vi "AssembleBLMultiplotScript-UandTI-CPPPNG.vi"(1 "Final Title":string, 2 "Spectra?":bool, 4 "Zref":dbl, 8 "Scale":dbl, 9 "BL Targets":T1[](array[typedef]) {"n" min=0.02 max=0.5 step=0.01 format="%.2f"}) -> (20 "gnuplotOut":string)   [LabVIEW 2021]
uses:
  BLTarget.ctl
  Results_plotter_Global.vi
panel:
  # "Currently displayed BL Target velocity profile will be overlaid"
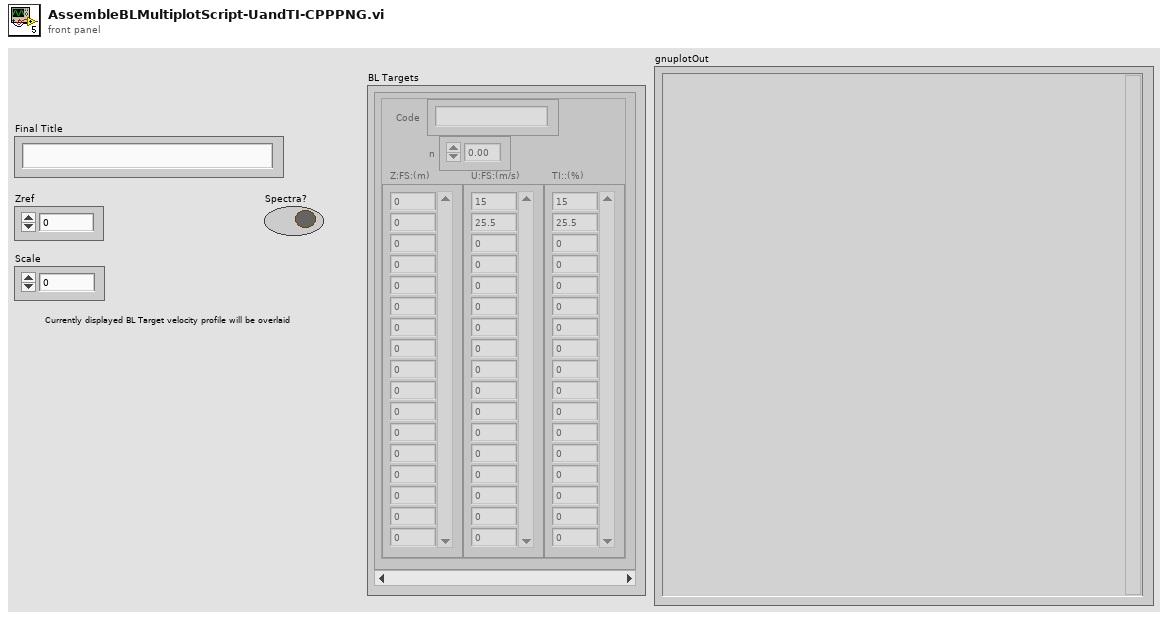
[diagram p1: front panel]
types:
  T1 = typedef "BLTarget.ctl" = cluster{"Code":string, "n":dbl, "Z:FS:(m)":dbl[], "U:FS:(m/s)":dbl[], "TI::(%)":dbl[]}
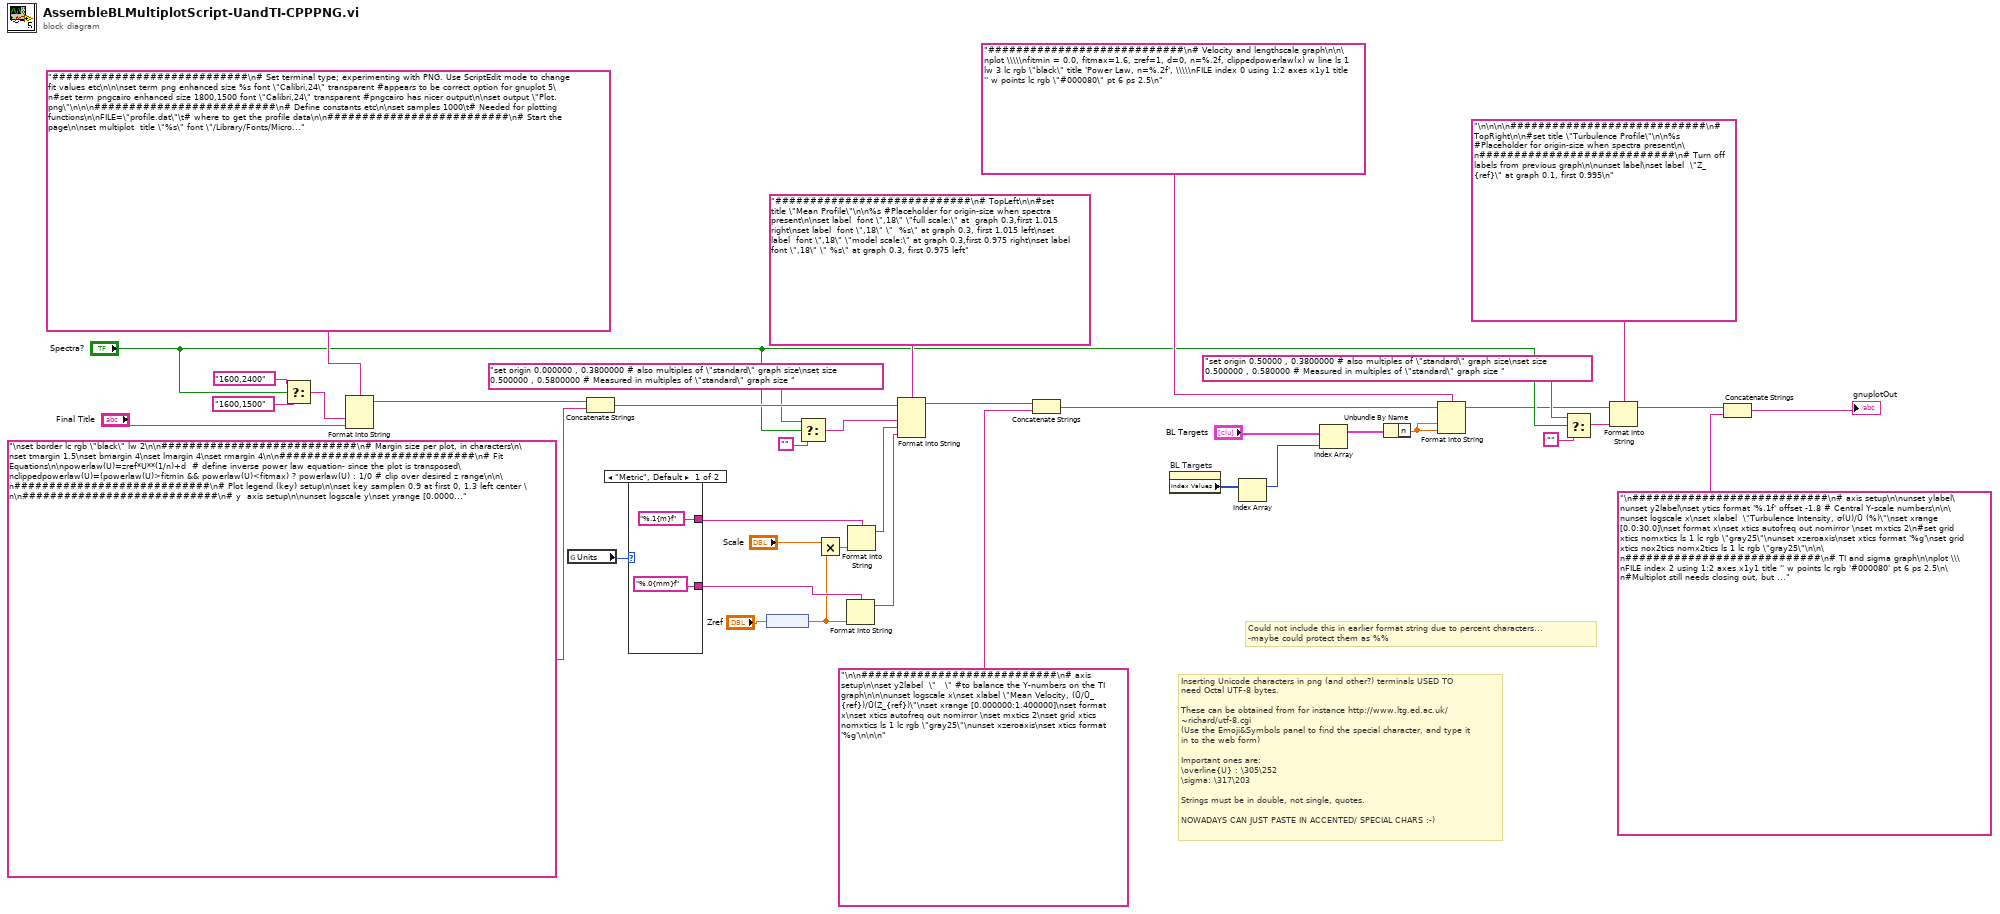
[diagram p0: block diagram]
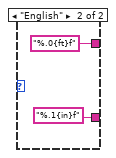
[diagram p2: hidden frame]
diagram:
  # "Could not include this in earlier format string due to percent characters...\n-maybe could protect them as %%"
  # "Inserting Unicode characters in png (and other?) terminals USED TO need Octal UTF-8 bytes. \n\nThese can be obtained from for instance http://www.ltg.ed.ac.uk/~richard/utf-8.cgi\n(Use the Emoji&Symbols panel to find the special character, and type it in to the web form)\n\nImportant ones are:\n\\overline{U} : \\305\\252\n\\sigma: \\317\\203\n\nStrings must be in double, not single, quotes.\n\nNOWADAYS CAN JUST PASTE IN ACCENTED/ SPECIAL CHARS :-)"
  n1 = Select(t="1600,2400", s="Spectra?", f="1600,1500") -> (s? t:f=w19:string)
  n2 = Format Into String(format string="############################\n# Set terminal type; experimenting with PNG. Use ScriptEdit mode to change fit values etc\n\n\nset term png enhanced size %s font \"Calibri,24\" transparent #appears to be correct option for gnuplot 5\n#set term pngcairo enhanced size 1800,1500 font \"Calibri,24\" transparent #pngcairo has nicer output\n\nset output \"Plot.png\"\n\n\n##########################\n# Define constants etc\n\nset samples 1000\t# Needed for plotting functions\n\nFILE=\"profile.dat\"\t# where to get the profile data\n\n##########################\n# Start the page\n\nset multiplot  title \"%s\" font \"/Library/Fonts/Microsoft/Calibri Bold.ttf, 32\" layout 1,2   #Note machine-dependent path\n", w19, "Final Title") -> (resulting string=w37:string)  [unwired: 2 in, 1 out]
  n3 = global read "Results_plotter_Global.vi" "Units"() -> (w2:enum16{"Metric", "English"})
  n4 = Concatenate Strings(w37, "\nset border lc rgb \"black\" lw 2\n\n############################\n# Margin size per plot, in characters\n\nset tmargin 1.5\nset bmargin 4\nset lmargin 4\nset rmargin 4\n\n############################\n# Fit Equations\n\npowerlaw(U)=zref*U**(1/n)+d  # define inverse power law equation- since the plot is transposed\nclippedpowerlaw(U)=(powerlaw(U)>fitmin && powerlaw(U)<fitmax) ? powerlaw(U) : 1/0 # clip over desired z range\n\n\n############################\n# Plot legend (key) setup\n\nset key samplen 0.9 at first 0, 1.3 left center \n\n############################\n# y  axis setup\n\nunset logscale y\nset yrange [0.000000:1.400]\nset mytics 2\nset grid ytics nomytics ls 1 lc rgb \"gray25\"\nunset yzeroaxis\nset ytics 0,0.2,1.4 in mirror format ''\n\nset label center at screen 0.5, first 0.925 \"Height\\n Z/Z_{ref}\"\n\n\n" ("string")) -> (w35:string)
  n5 = case shown="\"Metric\", Default" w2 {
    tunnel: ["%.1{m}f" ("format string") "%.0{ft}f" ("format string")] -> w4
    tunnel: ["%.0{mm}f" ("format string") "%.1{in}f" ("format string")] -> w3
    frame "Metric", Default {
    }
    frame "English" {
    }
  }
  n6 = node("Zref") -> (w1:dbl[unit])
  n7 = Select(t="set origin 0.000000 , 0.3800000 # also multiples of \"standard\" graph size\nset size 0.500000 , 0.5800000 # Measured in multiples of \"standard\" graph size ", s="Spectra?", f="") -> (s? t:f=w16:string)
  n8 = Multiply(x="Scale", y=w1) -> (x*y=w33:dbl[unit])
  n9 = Format Into String(format string=w3, w1) -> (resulting string=w5:string)  [unwired: 2 in, 1 out]
  n10 = Format Into String(format string=w4, w33) -> (resulting string=w6:string)  [unwired: 2 in, 1 out]
  n11 = Format Into String(format string="############################\n# TopLeft\n\n#set title \"Mean Profile\"\n\n%s #Placeholder for origin-size when spectra present\n\nset label  font \",18\" \"full scale:\" at  graph 0.3,first 1.015 right\nset label  font \",18\" \"  %s\" at graph 0.3, first 1.015 left\nset label  font \",18\" \"model scale:\" at graph 0.3,first 0.975 right\nset label  font \",18\" \" %s\" at graph 0.3, first 0.975 left", initial string=w35, w16, w6, w5) -> (resulting string=w36:string)  [unwired: 1 in, 1 out]
  n12 = Concatenate Strings(w36, "\n\n############################\n# axis setup\n\nset y2label  \"   \" #to balance the Y-numbers on the TI graph\n\n\nunset logscale x\nset xlabel \"Mean Velocity, (Ū/Ū_{ref})/Ū(Z_{ref})\"\nset xrange [0.000000:1.400000]\nset format x\nset xtics autofreq out nomirror \nset mxtics 2\nset grid xtics nomxtics ls 1 lc rgb \"gray25\"\nunset xzeroaxis\nset xtics format '%g'\n\n\n") -> (w30:string)
  n13 = property on="BL Targets" class="Arr (strict)"() -> ("Index Values"=w24:u32[])  [unwired: 2 in, 2 out]
  n14 = Index Array(array=w24) -> (element=w23:u32)  [unwired: 1 in]
  n15 = Index Array(array="BL Targets", index=w23) -> (element=w27:T1)
  n16 = Unbundle By Name(w27) -> ("n"=w26:dbl)
  n17 = Format Into String(format string="############################\n# Velocity and lengthscale graph\n\n\nplot \\\\\nfitmin = 0.0, fitmax=1.6, zref=1, d=0, n=%.2f, clippedpowerlaw(x) w line ls 1 lw 3 lc rgb \"black\" title 'Power Law, n=%.2f', \\\\\nFILE index 0 using 1:2 axes x1y1 title '' w points lc rgb \"#000080\" pt 6 ps 2.5\n", initial string=w30, w26, w26) -> (resulting string=w12:string)  [unwired: 1 in, 1 out]
  n18 = Select(t="set origin 0.50000 , 0.3800000 # also multiples of \"standard\" graph size\nset size 0.500000 , 0.580000 # Measured in multiples of \"standard\" graph size ", s="Spectra?", f="") -> (s? t:f=w10:string)
  n19 = Format Into String(format string="\n\n\n\n############################\n# TopRight\n\n#set title \"Turbulence Profile\"\n\n%s  #Placeholder for origin-size when spectra present\n\n############################\n# Turn off labels from previous graph\n\nunset label\nset label  \"Z_{ref}\" at graph 0.1, first 0.995\n", initial string=w12, w10) -> (resulting string=w11:string)  [unwired: 1 in, 1 out]
  n20 = Concatenate Strings(w11, "\n############################\n# axis setup\n\nunset ylabel\nunset y2label\nset ytics format '%.1f' offset -1.8 # Central Y-scale numbers\n\n\nunset logscale x\nset xlabel  \"Turbulence Intensity, σ(U)/Ū (%)\"\nset xrange [0.0:30.0]\nset format x\nset xtics autofreq out nomirror \nset mxtics 2\n#set grid xtics nomxtics ls 1 lc rgb \"gray25\"\nunset xzeroaxis\nset xtics format '%g'\nset grid xtics nox2tics nomx2tics ls 1 lc rgb \"gray25\"\n\n\n############################\n# TI and sigma graph\n\nplot \\\nFILE index 2 using 1:2 axes x1y1 title '' w points lc rgb '#000080' pt 6 ps 2.5\n\n#Multiplot still needs closing out, but that's handled by a later case...\n") -> (→"gnuplotOut":string)
